vi "RunQuestions(SubVI).vi"() -> ()   [LabVIEW 2013]
uses:
  FYP_LabviewGlobal(SubVI).vi
  <vilib>/addons/database/Connection.llb/DB Tools Open Connec (String).vi
  <vilib>/addons/database/_DB Variant To Data/Database Variant To Data.xnode
  <vilib>/addons/database/NI_Database_API.lvlib
panel:
  out "NoOfTrialsLeft":i32
  out "Time Stamp":timestamp format="%<%I:%M:%S %p\n%x>T"
  in  "Previous":bool
  in  "Next":bool
  out "QUESTION":i32
  # "Question:"
  # "You Still Left"
  # "Trials"
  # "Start Time:"
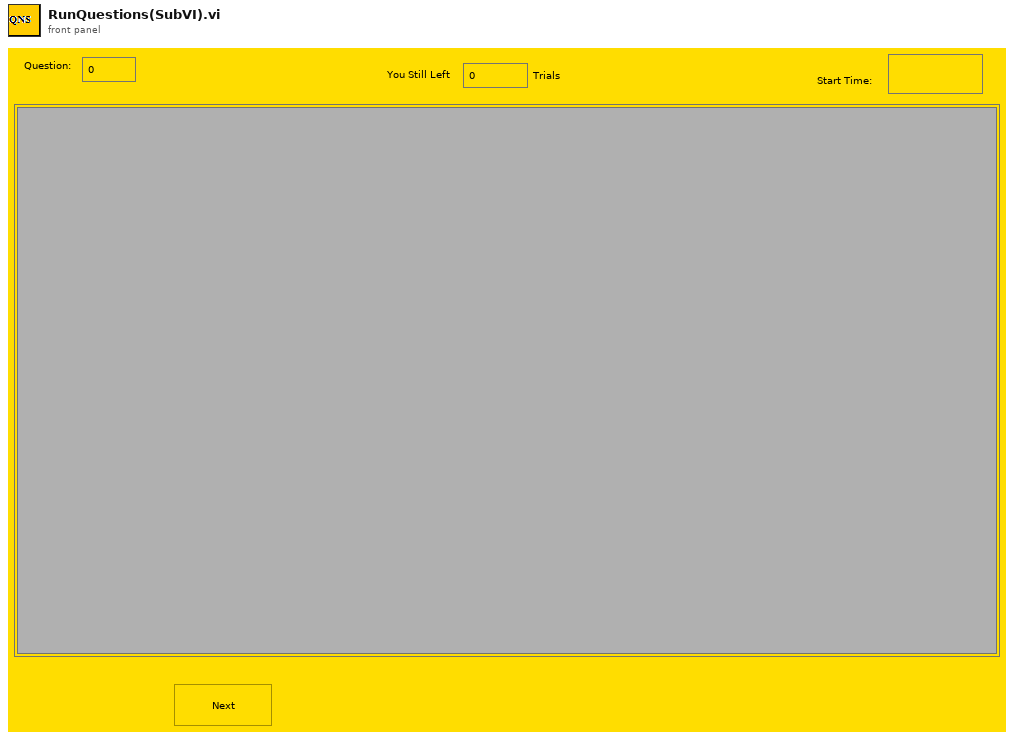
[diagram p1: front panel]
types:
  T1 = typedef "NI_Database_API.lvlib/Conn ObjectReference.ctl" = refnum<k1>
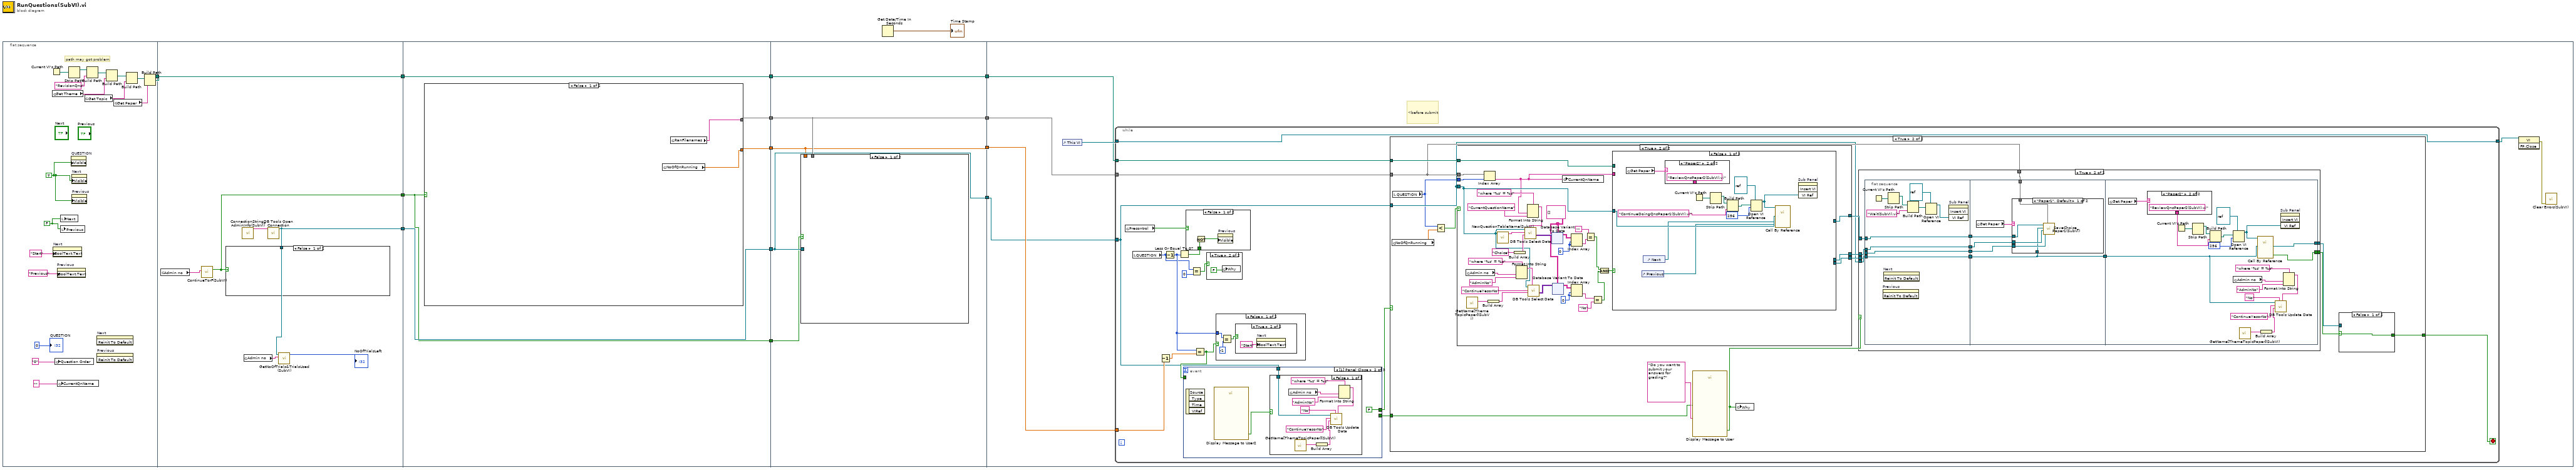
[diagram p0: block diagram]
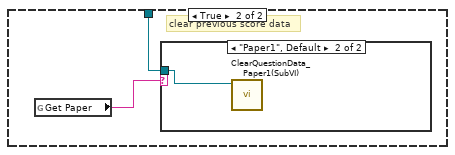
[diagram p2: hidden frame]
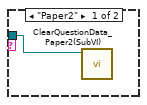
[diagram p3: hidden frame]
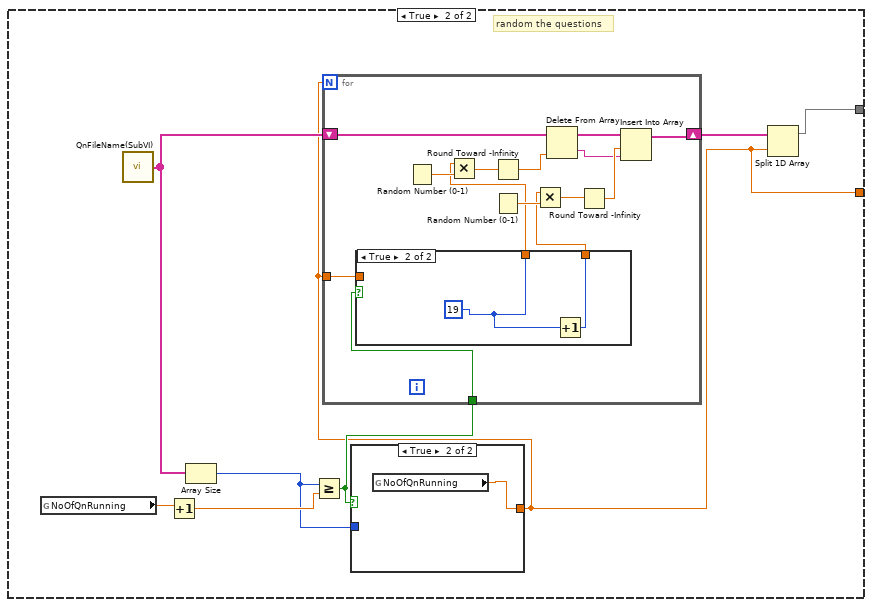
[diagram p4: hidden frame]
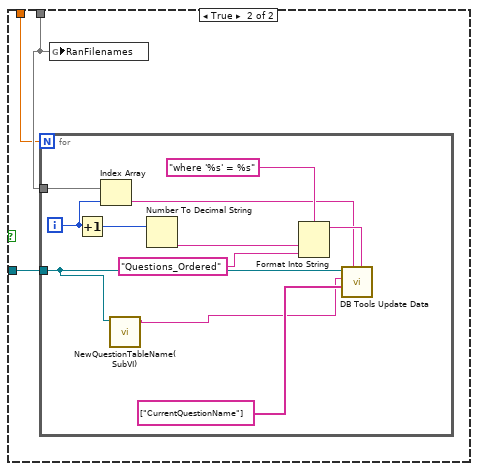
[diagram p7: hidden frame]
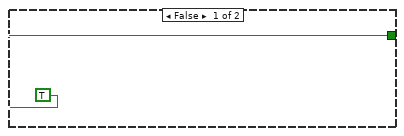
[diagram p8: hidden frame]
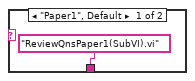
[diagram p10: hidden frame]
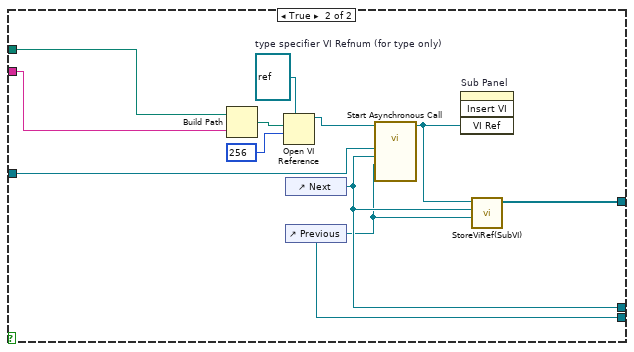
[diagram p11: hidden frame]
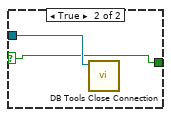
[diagram p12: hidden frame]
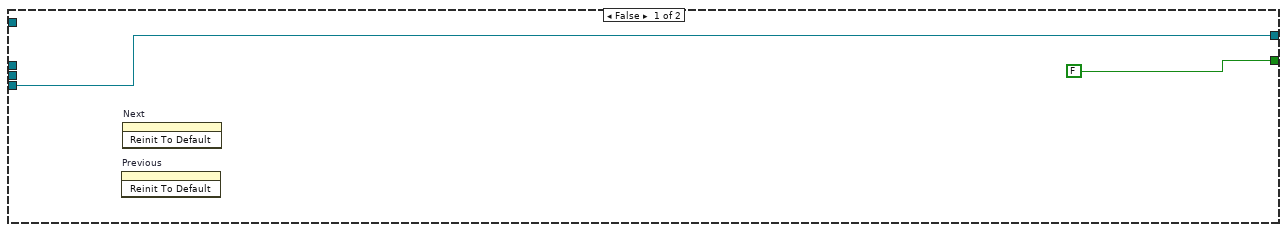
[diagram p13: hidden frame]
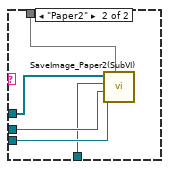
[diagram p14: hidden frame]
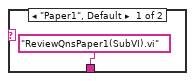
[diagram p15: hidden frame]
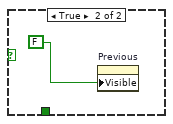
[diagram p16: hidden frame]
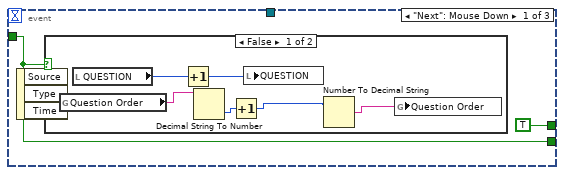
[diagram p17: hidden frame]
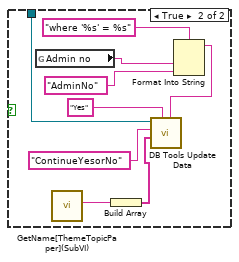
[diagram p19: hidden frame]
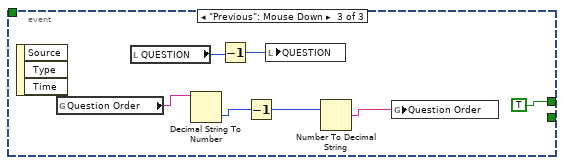
[diagram p20: hidden frame]
diagram:
  n1 = flat-sequence {
    tunnel: [w18] -> w13
    tunnel: w13 -> [w38]
    tunnel: [w38] -> w12
    tunnel: [w35] -> w11
    tunnel: [w33] -> w2
    tunnel: w12 -> [w47]
    tunnel: w11 -> [w45]
    tunnel: [w47] -> w10
    tunnel: [w46] -> w9
    tunnel: [w44] -> w8
    tunnel: [w45] -> w7
    tunnel: w2 -> [w43]
    tunnel: [w43] -> w1
    tunnel: w10 -> [w81]
    tunnel: w9 -> [w80]
    tunnel: w8 -> [w78]
    tunnel: w7 -> [w79]
    tunnel: [w81] -> w6
    tunnel: [w78] -> w5
    tunnel: [w80] -> w4
    tunnel: [w79] -> w3
    tunnel: w1 -> [w77]
    tunnel: w6 -> [w100]
    tunnel: w5 -> [w98]
    tunnel: w4 -> [w99]
    tunnel: w3 -> [w97]
    frame #0 {
      w20 = FALSE
      w21 = TRUE
      # "path may got problem"
      n2 = Current VI's Path() -> (path=w30:path)
      n3 = global read "FYP_LabviewGlobal(SubVI).vi" "Get Theme"() -> (w25:string)
      n4 = property on="Next" class="Bool (strict)"("BoolText.Text"="Start" ("Boolean Text.Text")) -> ()  [unwired: 2 in, 2 out]
      n5 = global write "FYP_LabviewGlobal(SubVI).vi" "Question Order"("0") -> ()
      n6 = property on="Previous" class="Bool (strict)"("BoolText.Text"="Previous" ("Boolean Text.Text")) -> ()  [unwired: 2 in, 2 out]
      n7 = global write "FYP_LabviewGlobal(SubVI).vi" "CurrentQnName"("") -> ()
      n8 = local write "Previous"(w20) -> ()
      n9 = local write "Next"(w20) -> ()
      n10 = Strip Path(path=w30) -> (stripped path=w29:path)  [unwired: 1 out]
      n11 = property on="QUESTION" class="DigNum (strict)"("Visible"=w21) -> ()  [unwired: 2 in, 2 out]
      n12 = property on="Next" class="Bool (strict)"("Visible"=w21) -> ()  [unwired: 2 in, 2 out]
      n13 = property on="Previous" class="Bool (strict)"("Visible"=w21) -> ()  [unwired: 2 in, 2 out]
      n14 = global read "FYP_LabviewGlobal(SubVI).vi" "Get Topic"() -> (w24:string)
      n15 = Build Path(base path=w29, name or relative path="RevisionQns") -> (appended path=w28:path)
      n16 = invoke on="Next" class="Bool (strict)" method="Reinit To Default"() -> ()  [unwired: 3 in, 3 out]
      n17 = invoke on="Previous" class="Bool (strict)" method="Reinit To Default"() -> ()  [unwired: 3 in, 3 out]
      n18 = Build Path(base path=w28, name or relative path=w25) -> (appended path=w27:path)
      n19 = global read "FYP_LabviewGlobal(SubVI).vi" "Get Paper"() -> (w22:string)
      n20 = Build Path(base path=w27, name or relative path=w24) -> (appended path=w23:path)
      n21 = Build Path(base path=w23, name or relative path=w22) -> (appended path=w18:path)
      "QUESTION" <- 0
    }
    frame #1 {
      n22 = global read "FYP_LabviewGlobal(SubVI).vi" "Admin no"() -> (w34:string)
      n23 = call "ContinueTorF(SubVI).vi"("AdminNo"=w34) -> ("Boolean"=w33:bool)  [unwired: 10 in]
      n24 = call "ConnectionString_AdminInfo(SubVI).vi"() -> ("ConnectionString"=w36:string)  [unwired: 11 in]
      n25 = global read "FYP_LabviewGlobal(SubVI).vi" "Admin no"() -> (w37:string)
      n26 = call-poly <vilib>:"DB Tools Open Connection.vi"("connection information"=w36) -> ("connection reference"=w35:T1)  [unwired: 7 in, 1 out]
      n27 = case shown="False" w33 {
        tunnel: w35 -> [_ w39]
        frame False {
        }
        frame True {
          # "clear previous score data"
          n28 = global read "FYP_LabviewGlobal(SubVI).vi" "Get Paper"() -> (w40:string)
          n29 = case shown="\"Paper1\", Default" w40 {
            tunnel: w39 -> [w41 w42]
            frame "Paper2" {
              n30 = call "ClearQuestionData_Paper2(SubVI).vi"("Refnum in"=w41) -> ()  [unwired: 11 in]
            }
            frame "Paper1", Default {
              n31 = call "ClearQuestionData_Paper1(SubVI).vi"("Refnum in"=w42) -> ()  [unwired: 11 in]
            }
          }
        }
      }
      n32 = call "GetNoOfTrials&TrialsUsed(SubVI).vi"("Admin no"=w37, "Refnum in"=w35) -> ("NoOfTrials"=→"NoOfTrialsLeft":i32)  [unwired: 8 in, 1 out]
    }
    frame #2 {
      n33 = case shown="False" w43 {
        tunnel: [w49 w50] -> w46
        tunnel: [w48 w51] -> w44
        frame False {
          n34 = global read "FYP_LabviewGlobal(SubVI).vi" "NoOfQnRunning"() -> (w48:dbl)
          n35 = global read "FYP_LabviewGlobal(SubVI).vi" "RanFilenames"() -> (w49:string[])
        }
        frame True {
          # "random the questions"
          n36 = global read "FYP_LabviewGlobal(SubVI).vi" "NoOfQnRunning"() -> (w56:dbl)
          n37 = call "QnFileName(SubVI).vi"() -> ("FileNames"=w55:string[])
          n38 = Increment(x=w56) -> (x+1=w57:dbl)
          n39 = Array Size(array=w55) -> (size(s)=w53:i32)
          n40 = Greater Or Equal?(x=w53, y=w57) -> (x >= y?=w54:bool)
          n41 = case shown="True" w54 {
            tunnel: [w58 w59] -> w51
            tunnel: w53 -> [w58 _]
            frame False {
            }
            frame True {
              n42 = global read "FYP_LabviewGlobal(SubVI).vi" "NoOfQnRunning"() -> (w59:dbl)
            }
          }
          n43 = for {
            N: w51 -> [_]
            shift-right: [w60] -> w52
            shift-left: w55 -> [w73]
            tunnel: w51 -> [w62]
            tunnel: w54 -> [w61]
            n44 = case shown="True" w61 {
              tunnel: [w74 w75] -> w64
              tunnel: [w74 w76] -> w63
              tunnel: w62 -> [w74 _]
              frame False {
              }
              frame True {
                w75 = 19
                n45 = Increment(x=w75) -> (x+1=w76:i32)
              }
            }
            n46 = Random Number (0-1)() -> (number: 0 to 1=w71:dbl)
            n47 = Multiply(x=w64, y=w71) -> (x*y=w70:dbl)
            n48 = Round Toward -Infinity(1:w70) -> (0:w69:dbl)
            n49 = Random Number (0-1)() -> (number: 0 to 1=w68:dbl)
            n50 = Multiply(x=w63, y=w68) -> (x*y=w67:dbl)
            n51 = Delete From Array(array=w73, index=w69) -> (deleted portion=w65:string, array with subset deleted=w72:string[])  [unwired: 1 in]
            n52 = Round Toward -Infinity(1:w67) -> (0:w66:dbl)
            n53 = Insert Into Array(array=w72, index=w66, new element=w65) -> (w60:string[])
          }
          n54 = Split 1D Array(array=w52, index=w51) -> (first subarray=w50:string[])  [unwired: 1 out]
        }
      }
    }
    frame #3 {
      n55 = case shown="False" w77 {
        tunnel: w80 -> [_ w84]
        tunnel: w79 -> [_ w83]
        tunnel: w78 -> [_ w82]
        frame False {
        }
        frame True {
          n56 = for {
            N: w82 -> [_]
            tunnel: w83 -> [w93]
            tunnel: w84 -> [w89]
            i -> [w85]
            n57 = Increment(x=w85) -> (x+1=w87:i32)
            n58 = Index Array(array=w89, index=w85) -> (element=w88:string)
            n59 = call "NewQuestionTableName(SubVI).vi"("connection reference"=w93) -> ("String"=w94:string)  [unwired: 9 in, 1 out]
            n60 = Number To Decimal String(number=w87) -> (decimal integer string=w86:string)  [unwired: 1 in]
            n61 = Format Into String(format string="where '%s' = %s", w86, "Questions_Ordered") -> (resulting string=w90:string)  [unwired: 2 in, 1 out]
            n62 = call <vilib>:"DB Tools Update Data.vi"("condition"=w90, "data"=w88, "columns"=string[] ["CurrentQuestionName"], "table"=w94, "connection reference"=w93) -> ()  [unwired: 5 in, 2 out]
          }
          n63 = global write "FYP_LabviewGlobal(SubVI).vi" "RanFilenames"(w84) -> ()
        }
      }
    }
    frame #4 {
      # "<before submit"
      n64 = control-ref of="This VI"() -> (w101:refnum<vi>)
      n65 = while {
        tunnel: w99 -> [w109]
        tunnel: w100 -> [w110]
        tunnel: w97 -> [w106]
        tunnel: w101 -> [w118]
        tunnel: [w118] -> w102
        tunnel: w98 -> [w107]
        stop <- w108 stop-if-true
        n66 = global read "FYP_LabviewGlobal(SubVI).vi" "Precontrol"() -> (w112:bool)
        n67 = local read "QUESTION"() -> (w104:i32)
        n68 = Decrement(x=w107) -> (x-1=w117:dbl)
        n69 = Decrement(x=w104) -> (x-1=w105:i32)
        n70 = Less Or Equal To 0?(x=w105) -> (x <= 0?=w113:bool)
        n71 = case shown="False" w112 {
          tunnel: w113 -> [w347 _]
          frame False {
            n72 = Not(x=w347) -> (.not. x?=w346:bool)
            n73 = property on="Previous" class="Bool (strict)"("Visible"=w346) -> ()  [unwired: 2 in, 2 out]
          }
          frame True {
            n74 = property on="Previous" class="Bool (strict)"("Visible"=FALSE) -> ()  [unwired: 2 in, 2 out]
          }
        }
        n75 = Equal?(x=w104, y=0) -> (x = y?=w115:bool)
        n76 = Equal?(x=w105, y=w117) -> (x = y?=w111:bool)
        n77 = event shown="[1] Panel Close" {
          selector: _ -> [_ _ _]
          dyn-events: _ -> [_ _ _]
          timeout: _ -> [_ _ _]
          tunnel: w111 -> [w350 _ _]
          tunnel: [w350 _ _] -> w114
          tunnel: [TRUE FALSE TRUE] -> w103
          tunnel: w106 -> [_ w357 _]
          event "Next": Mouse Down {
            n78 = event-data() -> ()  [unwired: 1 in, 3 out]
            n79 = case shown="False" w350 {
              frame False {
                n80 = global read "FYP_LabviewGlobal(SubVI).vi" "Question Order"() -> (w354:string)
                n81 = local read "QUESTION"() -> (w355:i32)
                n82 = Increment(x=w355) -> (x+1=w356:i32)
                n83 = Decimal String To Number(string=w354) -> (number=w353:i32)  [unwired: 2 in, 1 out]
                n84 = Increment(x=w353) -> (x+1=w352:i32)
                n85 = local write "QUESTION"(w356) -> ()
                n86 = Number To Decimal String(number=w352) -> (decimal integer string=w351:string)  [unwired: 1 in]
                n87 = global write "FYP_LabviewGlobal(SubVI).vi" "Question Order"(w351) -> ()
              }
              frame True {
              }
            }
          }
          event Panel Close {
            n88 = event-data() -> ()  [unwired: 1 in, 4 out]
            n89 = call "Display Message to User2"() -> ("OK"=w358:bool)  [unwired: 10 in, 1 out]
            n90 = case shown="False" w358 {
              tunnel: w357 -> [w360 w377]
              frame False {
                n91 = global read "FYP_LabviewGlobal(SubVI).vi" "Admin no"() -> (w364:string)
                n92 = call "GetName[ThemeTopicPaper](SubVI).vi"() -> ("Path for Score Table"=w363:string)  [unwired: 11 in]
                n93 = Build Array(w363) -> (w361:string[])
                n94 = Format Into String(format string="where '%s' = %s", w364, "AdminNo") -> (resulting string=w366:string)  [unwired: 2 in, 1 out]
                n95 = call <vilib>:"DB Tools Update Data.vi"("condition"=w366, "data"="No", "columns"=w361, "table"="ContinueYesorNo", "connection reference"=w360) -> ()  [unwired: 5 in, 2 out]
              }
              frame True {
                n96 = global read "FYP_LabviewGlobal(SubVI).vi" "Admin no"() -> (w372:string)
                n97 = call "GetName[ThemeTopicPaper](SubVI).vi"() -> ("Path for Score Table"=w371:string)  [unwired: 11 in]
                n98 = Build Array(w371) -> (w369:string[])
                n99 = Format Into String(format string="where '%s' = %s", w372, "AdminNo") -> (resulting string=w374:string)  [unwired: 2 in, 1 out]
                n100 = call <vilib>:"DB Tools Update Data.vi"("condition"=w374, "data"="Yes", "columns"=w369, "table"="ContinueYesorNo", "connection reference"=w377) -> ()  [unwired: 5 in, 2 out]
              }
            }
          }
          event "Previous": Mouse Down {
            n101 = event-data() -> ()  [unwired: 1 in, 3 out]
            n102 = global read "FYP_LabviewGlobal(SubVI).vi" "Question Order"() -> (w382:string)
            n103 = local read "QUESTION"() -> (w383:i32)
            n104 = Decimal String To Number(string=w382) -> (number=w380:i32)  [unwired: 2 in, 1 out]
            n105 = Decrement(x=w383) -> (x-1=w384:i32)
            n106 = Decrement(x=w380) -> (x-1=w379:i32)
            n107 = local write "QUESTION"(w384) -> ()
            n108 = Number To Decimal String(number=w379) -> (decimal integer string=w381:string)  [unwired: 1 in]
            n109 = global write "FYP_LabviewGlobal(SubVI).vi" "Question Order"(w381) -> ()
          }
        }
        n110 = case shown="True" w115 {
          frame False {
          }
          frame True {
            n111 = global write "FYP_LabviewGlobal(SubVI).vi" "Why"(FALSE) -> ()
          }
        }
        n112 = case shown="False" w111 {
          tunnel: w105 -> [w386 _]
          frame False {
            n113 = Equal?(x=w386, y=-1) -> (x = y?=w385:bool)
            n114 = case shown="True" w385 {
              frame False {
                n115 = property on="Next" class="Bool (strict)"("BoolText.Text"="Next" ("Boolean Text.Text")) -> ()  [unwired: 2 in, 2 out]
              }
              frame True {
                n116 = property on="Next" class="Bool (strict)"("BoolText.Text"="Start" ("Boolean Text.Text")) -> ()  [unwired: 2 in, 2 out]
              }
            }
          }
          frame True {
            n117 = property on="Next" class="Bool (strict)"("BoolText.Text"="End") -> ()  [unwired: 2 in, 2 out]
          }
        }
        n118 = case shown="True" w103 {
          tunnel: w114 -> [_ w133]
          tunnel: w110 -> [_ w131]
          tunnel: w109 -> [_ w130]
          tunnel: [TRUE w124] -> w108
          tunnel: w106 -> [_ w123]
          frame False {
          }
          frame True {
            n119 = global read "FYP_LabviewGlobal(SubVI).vi" "NoOfQnRunning"() -> (w122:dbl)
            n120 = local read "QUESTION"() -> (w120:i32)
            n121 = Less?(x=w120, y=w122) -> (x < y?=w121:bool)
            n122 = case shown="True" w121 {
              tunnel: w120 -> [_ w160]
              tunnel: w131 -> [_ w169]
              tunnel: w130 -> [_ w161]
              tunnel: [_ w168] -> w129
              tunnel: [_ w167] -> w128
              tunnel: [_ w166] -> w127
              tunnel: w123 -> [_ w148]
              frame False {
              }
              frame True {
                w141 = 0 ("disabled index (col)")
                w155 = 0 ("disabled index (col)")
                w143 = string[][] []
                n123 = global read "FYP_LabviewGlobal(SubVI).vi" "Admin no"() -> (w150:string)
                n124 = call "GetName[ThemeTopicPaper](SubVI).vi"() -> ("Path for Score Table"=w146:string)  [unwired: 11 in]
                n125 = Index Array(array=w161, index=w160) -> (element=w135:string)
                n126 = Build Array(w146) -> (w145:string[])
                n127 = call "NewQuestionTableName(SubVI).vi"("connection reference"=w148) -> ("String"=w164:string)  [unwired: 9 in, 1 out]
                n128 = Build Array("Choice") -> (w162:string[])
                n129 = Format Into String(format string="where '%s' = %s", w150, "AdminNo") -> (resulting string=w149:string)  [unwired: 2 in, 1 out]
                n130 = Format Into String(format string="where '%s' = %s", w135, "CurrentQuestionName") -> (resulting string=w157:string)  [unwired: 2 in, 1 out]
                n131 = call <vilib>:"DB Tools Select Data.vi"("condition"=w157, "columns"=w162, "table"=w164, "connection reference"=w148) -> ("data"=w165:variant[][])  [unwired: 2 in, 2 out]
                n132 = call <vilib>:"DB Tools Select Data.vi"("condition"=w149, "columns"=w145, "table"="ContinueYesorNo", "connection reference"=w148) -> ("data"=w144:variant[][])  [unwired: 2 in, 2 out]
                n133 = xnode "Database Variant To Data"("database variant"=w165, "type"=w143) -> ("data"=w156:string[][])  [unwired: 1 in, 1 out]
                n134 = xnode "Database Variant To Data"("database variant"=w144, "type"=w143) -> ("data"=w142:string[][])  [unwired: 1 in, 1 out]
                n135 = global write "FYP_LabviewGlobal(SubVI).vi" "CurrentQnName"(w135) -> ()
                n136 = Index Array(array=w156, index (row)=w155, index (col)=w155) -> (element=w153:string)
                n137 = Index Array(array=w142, index (row)=w141, index (col)=w141) -> (element=w139:string)
                n138 = Equal?(x="", y=w153) -> (x = y?=w138:bool)
                n139 = Equal?(x=w139, y="No") -> (x = y?=w137:bool)
                n140 = And(x=w138, y=w137) -> (x .and. y?=w136:bool)
                n141 = case shown="False" w136 {
                  tunnel: w169 -> [_ w277]
                  tunnel: [_ w275] -> w168
                  tunnel: [_ w274] -> w167
                  tunnel: [_ w273] -> w166
                  tunnel: w148 -> [w260 w272]
                  tunnel: w135 -> [_ w271]
                  frame False {
                    n142 = global read "FYP_LabviewGlobal(SubVI).vi" "Get Paper"() -> (w262:string)
                    n143 = control-ref of="Previous"() -> (w258:refnum<vi>)
                    n144 = control-ref of="Next"() -> (w259:refnum<vi>)
                    n145 = case shown="\"Paper2\"" w262 {
                      tunnel: ["ReviewQnsPaper1(SubVI).vi" ("name or relative path") "ReviewQnsPaper2(SubVI).vi" ("name or relative path")] -> _
                      frame "Paper1", Default {
                      }
                      frame "Paper2" {
                      }
                    }
                    n146 = Current VI's Path() -> (path=w268:path)
                    n147 = Strip Path(path=w268) -> (stripped path=w267:path)  [unwired: 1 out]
                    n148 = Build Path(base path=w267, name or relative path="ContinueDoingQnsPaper1(SubVI).vi") -> (appended path=w265:path)
                    n149 = Open VI Reference(type specifier VI Refnum (for type only)=refnum<vi> refnum, vi path=w265, options=256) -> (vi reference=w263:refnum<vi>)  [unwired: 3 in, 1 out]
                    n150 = call-by-ref "?"(reference=w263, "RefPrevious"=w258, "RefNext"=w259, "connection reference"=w260) -> ()  [unwired: 10 in, 2 out]
                    n151 = invoke on="Sub Panel" class="SubPnl" method="Insert VI"("VI Ref"=w263) -> ()  [unwired: 3 in, 4 out]
                  }
                  frame True {
                    w280 = refnum<vi> refnum  # type specifier VI Refnum (for type only)
                    n152 = Build Path(base path=w277, name or relative path=w271) -> (appended path=w278:path)
                    n153 = Open VI Reference(type specifier VI Refnum (for type only)=w280, vi path=w278, options=256) -> (vi reference=w279:refnum<vi>)  [unwired: 3 in, 1 out]
                    n154 = control-ref of="Next"() -> (w274:refnum<vi>)
                    n155 = control-ref of="Previous"() -> (w273:refnum<vi>)
                    n156 = call-by-ref "Start Asynchronous Call"(reference=w279, "RefPrevious"=w273, "RefNext"=w274, "connection reference"=w272) -> (reference out=w276:refnum<vi>)  [unwired: 9 in, 2 out]
                    n157 = invoke on="Sub Panel" class="SubPanel" method="Insert VI"("VI Ref"=w276) -> ()  [unwired: 3 in, 4 out]
                    n158 = call "StoreViRef(SubVI).vi"("Previous 2"=w273, "Next 2"=w274, "vi reference"=w276) -> ("Array"=w275:refnum<vi>[])  [unwired: 8 in]
                  }
                }
              }
            }
            n159 = call "Display Message to User"("Enable"=w133, "Message"="Do you want to submit your answers for grading?") -> ("OK"=w132:bool)  [unwired: 8 in, 1 out]
            n160 = global write "FYP_LabviewGlobal(SubVI).vi" "Why"(w132) -> ()
            n161 = case shown="True" w132 {
              tunnel: w123 -> [w286 w298]
              tunnel: [FALSE w296] -> w125
              tunnel: [w286 w297] -> w126
              tunnel: w129 -> [_ w293]
              tunnel: w128 -> [_ w291]
              tunnel: w127 -> [_ w289]
              tunnel: w130 -> [_ w287]
              frame False {
                n162 = invoke on="Previous" class="Bool (strict)" method="Reinit To Default"() -> ()  [unwired: 3 in, 3 out]
                n163 = invoke on="Next" class="Bool (strict)" method="Reinit To Default"() -> ()  [unwired: 3 in, 3 out]
              }
              frame True {
                n164 = flat-sequence {
                  tunnel: [w308] -> w295
                  tunnel: w298 -> [w308]
                  tunnel: w293 -> [w301]
                  tunnel: [w301] -> w292
                  tunnel: w291 -> [w300]
                  tunnel: [w300] -> w290
                  tunnel: w289 -> [w299]
                  tunnel: [w299] -> w288
                  tunnel: w295 -> [w310]
                  tunnel: [w310] -> w294
                  tunnel: w292 -> [w313]
                  tunnel: w290 -> [w312]
                  tunnel: w288 -> [w311]
                  tunnel: w287 -> [w309]
                  tunnel: w294 -> [w326]
                  tunnel: [w325] -> w296
                  tunnel: [w338] -> w297
                  frame #0 {
                    n165 = Current VI's Path() -> (path=w307:path)
                    n166 = invoke on="Previous" class="Bool (strict)" method="Reinit To Default"() -> ()  [unwired: 3 in, 3 out]
                    n167 = invoke on="Next" class="Bool (strict)" method="Reinit To Default"() -> ()  [unwired: 3 in, 3 out]
                    n168 = Strip Path(path=w307) -> (stripped path=w306:path)  [unwired: 1 out]
                    n169 = Build Path(base path=w306, name or relative path="Wait(SubVI).vi") -> (appended path=w304:path)
                    n170 = Open VI Reference(type specifier VI Refnum (for type only)=refnum<vi> refnum, vi path=w304) -> (vi reference=w302:refnum<vi>)  [unwired: 4 in, 1 out]
                    n171 = invoke on="Sub Panel" class="SubPnl" method="Insert VI"("VI Ref"=w302) -> ()  [unwired: 3 in, 4 out]
                  }
                  frame #1 {
                    n172 = global read "FYP_LabviewGlobal(SubVI).vi" "Get Paper"() -> (w314:string)
                    n173 = case shown="\"Paper1\", Default" w314 {
                      tunnel: w313 -> [w319 w324]
                      tunnel: w312 -> [w318 w323]
                      tunnel: w311 -> [w317 w322]
                      tunnel: w310 -> [w316 w321]
                      tunnel: w309 -> [w315 w320]
                      frame "Paper1", Default {
                        n174 = call "SaveChoice_Paper1(SubVI).vi"("RanFilenames"=w315, "Previous 2"=w317, "Next 2"=w318, "connection reference"=w316, "Array"=w319) -> ()  [unwired: 7 in]
                      }
                      frame "Paper2" {
                        n175 = call "SaveImage_Paper2(SubVI).vi"("RanFilenames"=w320, "Previous 2"=w322, "Next 2"=w323, "connection reference"=w321, "Array"=w324) -> ()  [unwired: 7 in]
                      }
                    }
                  }
                  frame #2 {
                    n176 = global read "FYP_LabviewGlobal(SubVI).vi" "Get Paper"() -> (w335:string)
                    n177 = case shown="\"Paper2\"" w335 {
                      tunnel: ["ReviewQnsPaper1(SubVI).vi" ("name or relative path") "ReviewQnsPaper2(SubVI).vi" ("name or relative path")] -> w336
                      frame "Paper1", Default {
                      }
                      frame "Paper2" {
                      }
                    }
                    n178 = Current VI's Path() -> (path=w343:path)
                    n179 = Strip Path(path=w343) -> (stripped path=w342:path)  [unwired: 1 out]
                    n180 = Build Path(base path=w342, name or relative path=w336) -> (appended path=w340:path)
                    n181 = Open VI Reference(type specifier VI Refnum (for type only)=refnum<vi> refnum, vi path=w340, options=256) -> (vi reference=w337:refnum<vi>)  [unwired: 3 in, 1 out]
                    n182 = global read "FYP_LabviewGlobal(SubVI).vi" "Admin no"() -> (w330:string)
                    n183 = call "GetName[ThemeTopicPaper](SubVI).vi"() -> ("Path for Score Table"=w329:string)  [unwired: 11 in]
                    n184 = call-by-ref "?"(reference=w337, "connection reference"=w326) -> ("Close?"=w325:bool, "connection reference out"=w338:T1)  [unwired: 10 in, 2 out]
                    n185 = Build Array(w329) -> (w327:string[])
                    n186 = invoke on="Sub Panel" class="SubPnl" method="Insert VI"("VI Ref"=w337) -> ()  [unwired: 3 in, 4 out]
                    n187 = Format Into String(format string="where '%s' = %s", w330, "AdminNo") -> (resulting string=w332:string)  [unwired: 2 in, 1 out]
                    n188 = call <vilib>:"DB Tools Update Data.vi"("condition"=w332, "data"="No", "columns"=w327, "table"="ContinueYesorNo", "connection reference"=w326) -> ()  [unwired: 5 in, 2 out]
                  }
                }
              }
            }
            n189 = case shown="False" w125 {
              selector: w125 -> [w282 w283]
              tunnel: w126 -> [_ w284]
              tunnel: [w282 w283] -> w124
              frame False {
              }
              frame True {
                n190 = call <vilib>:"DB Tools Close Connection.vi"("connection reference"=w284) -> ()  [unwired: 6 in, 1 out]
              }
            }
          }
        }
      }
      n191 = invoke class="VI" method="FP.Close"(reference=w102) -> (error out=w96:errorcluster)  [unwired: 2 in, 2 out]
      n192 = call "Clear Errors(SubVI).vi"("error in (no error)"=w96) -> ()  [unwired: 6 in, 1 out]
    }
  }
  n193 = Get Date/Time In Seconds() -> (seconds since 1Jan1904=→"Time Stamp":timestamp)
